vi "test_Multiple Global Enum with Format and Type Cast Array Command Messages using Trigger and Protection.vi"(8 "error in (no error)":errorcluster, 11 "TestCase in":refnum<class "Instrument Addon Common System Tests.lvclass">) -> (0 "error out":errorcluster, 3 "TestCase out":refnum<class "Instrument Addon Common System Tests.lvclass">)   [LabVIEW 2019, in "Instrument Addon Common System Tests.lvclass"]
uses:
  Instrument Addon Common System Tests.lvclass
  <vilib>/addons/_JKI Toolkits/VI Tester/TestCase.llb/TestCase.lvclass
  <vilib>/NI VeriStand/Execution/Workspace/NI_VS Workspace ExecutionAPI.lvlib
  <vilib>/NI VeriStand/Execution/Workspace/NI VeriStand - Get Multiple Channel Values.vi
  <vilib>/NI VeriStand/Execution/Workspace/NI VeriStand - Set Multiple Channel Values.vi
  C:/Users/nitest/Desktop/Git 2019/niveristand-custom-device-testing-tools/VeriStandTestCase/VeriStandTestCase.lvclass
  C:/Program Files (x86)/National Instruments/LabVIEW 2019/vi.lib/addons/_JKI Toolkits/VI Tester/TestCase.llb/TestCase.lvclass
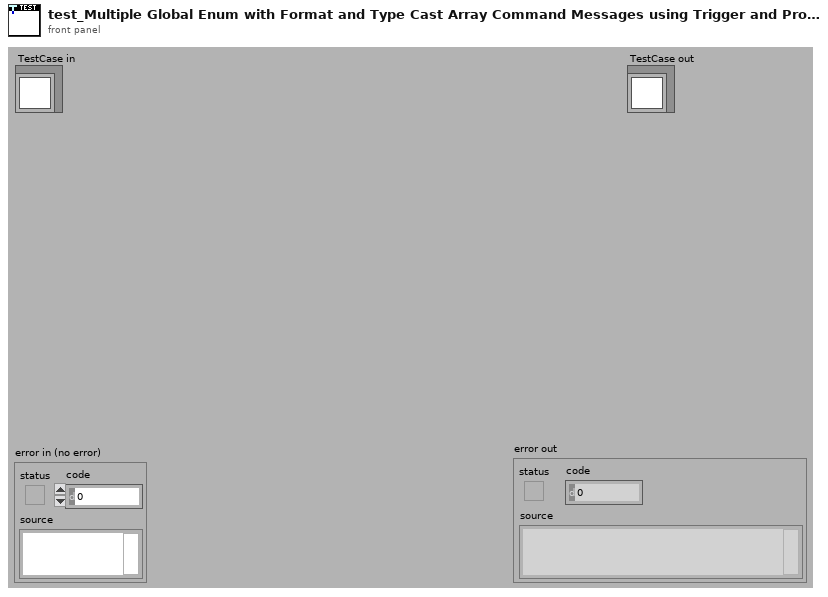
[diagram p1: front panel]
types:
  T1 = typedef "NI_VS Workspace ExecutionAPI.lvlib/WorkspaceAPI.ctl" = refnum<k24>
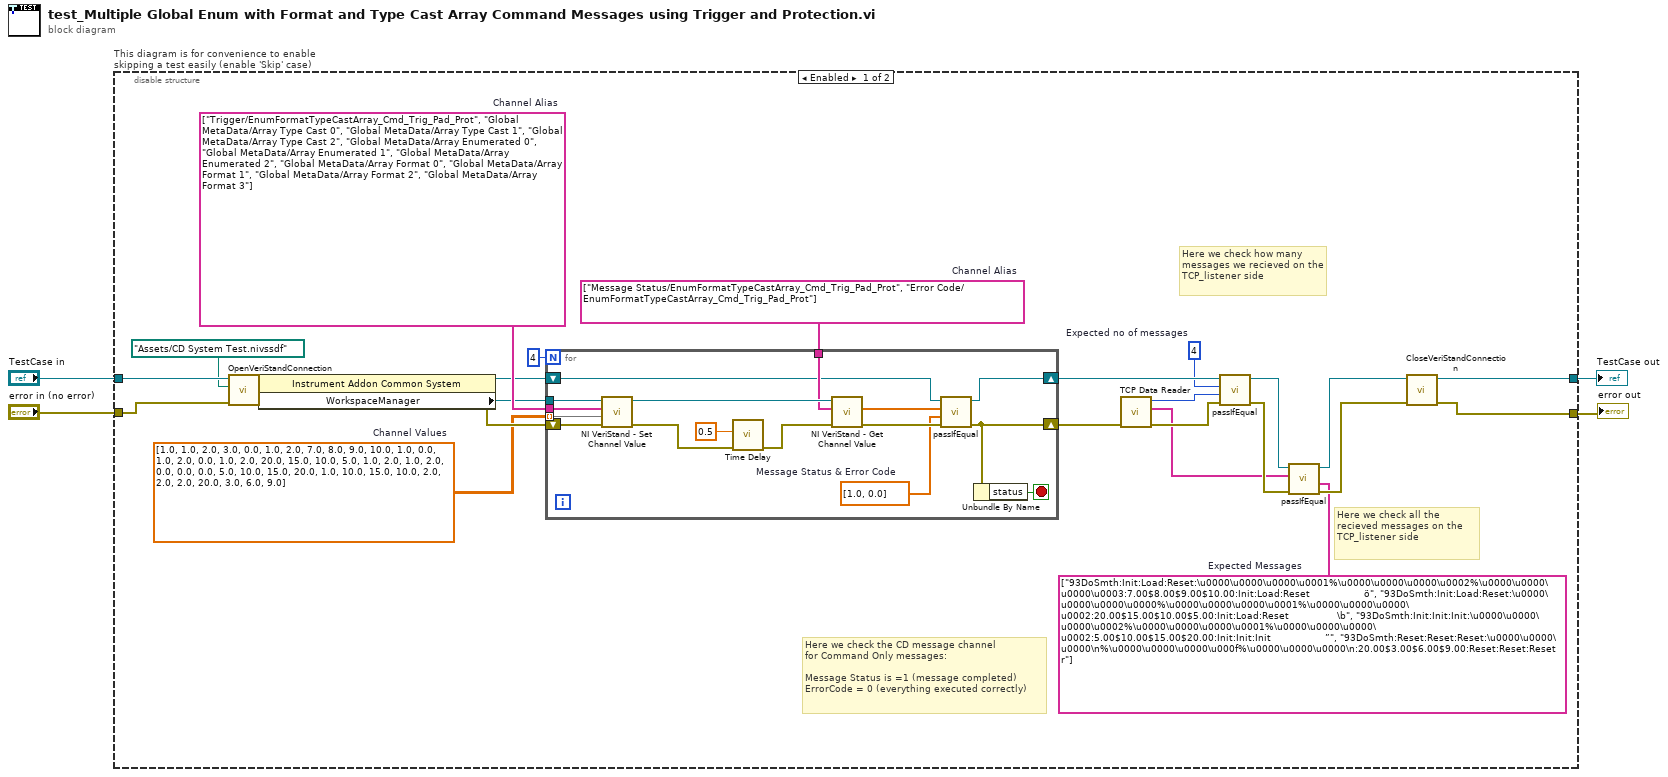
[diagram p0: block diagram]
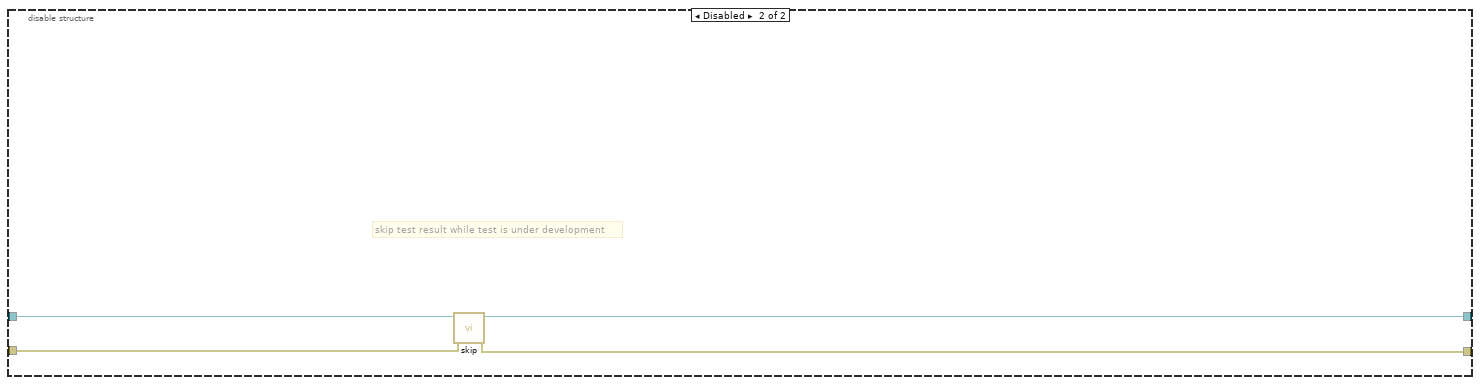
[diagram p2: hidden frame]
diagram:
  n1 = disable-structure "This diagram is for convenience to enable skipping a test easily (enable 'Skip' case)" shown="Enabled" {
    disable-tunnel: "TestCase in" -> [w27 w49]
    disable-tunnel: [w28 w47] -> w1
    disable-tunnel: [w29 w48] -> w3
    disable-tunnel: "error in (no error)" -> [w25 w46]
    frame Enabled {
      w5 = string[] ["93DoSmth:Init:Load:Reset:\u0000\u0000\u0000\u0001%\u0000\u0000\u0000\u0002%\u0000\u0000\u0000\u0003:7.00$8.00$9.00$10.00:Init:Load:Reset                  ö", "93DoSmth:Init:Load:Reset:\u0000\u0000\u0000\u0000%\u0000\u0000\u0000\u0001%\u0000\u0000\u0000\u0002:20.00$15.00$10.00$5.00:Init:Load:Reset                \b", "93DoSmth:Init:Init:Init:\u0000\u0000\u0000\u0002%\u0000\u0000\u0000\u0001%\u0000\u0000\u0000\u0002:5.00$10.00$15.00$20.00:Init:Init:Init                  ”", "93DoSmth:Reset:Reset:Reset:\u0000\u0000\u0000\n%\u0000\u0000\u0000\u000f%\u0000\u0000\u0000\n:20.00$3.00$6.00$9.00:Reset:Reset:Reset              r"]  # Expected Messages
      w8 = 4  # Expected no of messages
      w17 = string[] ["Message Status/EnumFormatTypeCastArray_Cmd_Trig_Pad_Prot", "Error Code/EnumFormatTypeCastArray_Cmd_Trig_Pad_Prot"]  # Channel Alias
      w20 = dbl[][] [[1.0, 1.0, 2.0, 3.0, 0.0, 1.0, 2.0, 7.0, 8.0, 9.0, 10.0], [1.0, 0.0, 1.0, 2.0, 0.0, 1.0, 2.0, 20.0, 15.0, 10.0, 5.0], [1.0, 2.0, 1.0, 2.0, 0.0, 0.0, 0.0, 5.0, 10.0, 15.0, 20.0], [1.0, 10.0, 15.0, 10.0, 2.0, 2.0, 2.0, 20.0, 3.0, 6.0, 9.0]]  # Channel Values
      w21 = string[] ["Trigger/EnumFormatTypeCastArray_Cmd_Trig_Pad_Prot", "Global MetaData/Array Type Cast 0", "Global MetaData/Array Type Cast 1", "Global MetaData/Array Type Cast 2", "Global MetaData/Array Enumerated 0", "Global MetaData/Array Enumerated 1", "Global MetaData/Array Enumerated 2", "Global MetaData/Array Format 0", "Global MetaData/Array Format 1", "Global MetaData/Array Format 2", "Global MetaData/Array Format 3"]  # Channel Alias
      # "Here we check how many messages we recieved on the TCP_listener side"
      # "Here we check all the recieved messages on the TCP_listener side"
      # "Here we check the CD message channel\nfor Command Only messages:\n\nMessage Status is =1 (message completed)\nErrorCode = 0 (everything executed correctly)"
      n2 = call-dynamic "OpenVeriStandConnection.vi"("error in (no error)"=w25, "System Definition File"=path "Assets/CD System Test.nivssdf", "VeriStand Test Case in"=w27) -> ("error out"=w24:errorcluster, "VeriStand Test Case out"=w26:refnum<class "Instrument Addon Common System Tests.lvclass">)  [unwired: 6 in, 1 out]
      n3 = property class="Instrument Addon Common System "(reference=w26, error in=w24) -> (reference out=w18:refnum<class "Instrument Addon Common System Tests.lvclass">, error out=w22:errorcluster, "WorkspaceManager"=w16:T1)
      n4 = for {
        N: 4 -> [_]
        tunnel: w16 -> [w45]
        tunnel: w21 -> [w43]
        tunnel: w20 -> [w42] mode=indexing
        shift-right: [w31] -> w7
        shift-left: w22 -> [w44]
        tunnel: w17 -> [w40]
        shift-right: [w35] -> w15
        shift-left: w18 -> [w36]
        stop <- w30 stop-if-true
        w32 = dbl[] [1.0, 0.0]  # Message Status & Error Code
        n5 = call-poly <vilib>:"NI VeriStand - Set Channel Value.vi"("error in (no error)"=w44, "Values"=w42, "Channels"=w43, "WorkspaceManager in"=w45) -> ("error out"=w38:errorcluster, "WorkspaceManager out"=w41:T1)  [unwired: 6 in]
        n6 = call "Time Delay"("error in (no error)"=w38, "Delay Time (s)"=0.5) -> ("error out"=w37:errorcluster)  [unwired: 9 in]
        n7 = call-poly <vilib>:"NI VeriStand - Get Channel Value.vi"("error in (no error)"=w37, "Channels"=w40, "WorkspaceManager in"=w41) -> ("error out"=w34:errorcluster, "Values"=w33:dbl[])  [unwired: 6 in, 1 out]
        n8 = call-dynamic "passIfEqual.vi"("error in (no error)"=w34, "y"=w32, "x"=w33, "TestCase in"=w36) -> ("error out"=w31:errorcluster, "TestCase out"=w35:refnum<class "Instrument Addon Common System Tests.lvclass">)  [unwired: 6 in]
        n9 = Unbundle By Name(w31) -> ("status"=w30:bool)
      }
      n10 = call "TCP Data Reader.vi"("error in (no error)"=w7) -> ("error out"=w13:errorcluster, "Recieved Messages"=w6:string[], "No of messages"=w9:i32)  [unwired: 8 in]
      n11 = call-dynamic "passIfEqual.vi"("error in (no error)"=w13, "y"=w9, "x"=w8, "TestCase in"=w15) -> ("error out"=w11:errorcluster, "TestCase out"=w14:refnum<class "Instrument Addon Common System Tests.lvclass">)  [unwired: 6 in]
      n12 = call-dynamic "passIfEqual.vi"("error in (no error)"=w11, "y"=w5, "x"=w6, "TestCase in"=w14) -> ("error out"=w10:errorcluster, "TestCase out"=w12:refnum<class "Instrument Addon Common System Tests.lvclass">)  [unwired: 6 in]
      n13 = call-dynamic "CloseVeriStandConnection.vi"("error in (no error)"=w10, "VeriStand Test Case in"=w12) -> ("error out"=w29:errorcluster, "VeriStand Test Case out"=w28:refnum<class "Instrument Addon Common System Tests.lvclass">)  [unwired: 8 in]
    }
    frame Disabled {
      # "skip test result while test is under development"
      n14 = call <vilib>:"skip.vi"("error in (no error)"=w46, "TestCase in"=w49) -> ("error out"=w48:errorcluster, "TestCase out"=w47:refnum<class "Instrument Addon Common System Tests.lvclass">)  [unwired: 8 in]
    }
  }
  "error out" <- w3
  "TestCase out" <- w1
